vi "calculateSpectra.vi"(8 "ErrorIn":errorcluster, 10 "Tacho signal In":waveform(dbl), 11 "AccelerationDataIn":waveform(dbl)[](array[waveform])) -> (0 "ErrorOut":errorcluster, 1 "Rotational speed [RPM]":dbl format="%0.2f", 2 "AccelerationDataFrames":T8, 3 "AccelerationDataOut":waveform(dbl)[](array[waveform]), 4 "order power spectra":T7(array[cluster]) {"order 0" format="%.2p"; "delta order" format="%.2p"; "magnitude" format="%.2f"}, 5 "Tacho signal out":waveform(dbl), 6 "spectrum info":T1[](array[typedef]) {"x-axis units" items=["Time (s)"=0, "Frequency-CB (Hz)"=1, "Frequency-CPB (Hz)"=1248, "Frequency-Arbitrary (Hz)"=2357, "Quefrency (s)"=2, "Revolutions (rev)"=3, "Order"=4, "Speed (RPM)"=11, "Speed (rad/s)"=21, "Index"=65535]; "weighting filter" items=["Linear", "A-weighting", "B-weighting", "C-weighting", "ITU-R 468-4", "Dolby", "CCITT", "C-message", "Wb", "Wc", "Wd", "We", "Wf", "Wh", "Wj", "Wk", "Wm", "AES17 20 kHz lowpass", "AES17 40 kHz lowpass", "AES17 20 kHz highpass", "AES17 40 kHz highpass"]; "dB reference [EU]" format="%.2f"; "engineering units" items=["custom..."=0, "V"=1, "A"=21, "C"=30, "pC"=31, "s"=32, "-"=29, "Pa"=2, "N"=20, "g"=3, "m/s^2"=4, "m/s"=5, "m"=6, "mm/s"=12, "mm"=13, "micron/s"=14, "micron"=15, "in/s^2"=7, "in/s"=8, "in"=9, "mil/s"=10, "mil"=11, "rad/s^2"=16, "rad/s"=17, "rad"=18, "deg/s^2"=26, "deg/s"=27, "deg"=28, "RPM"=22, "cycle/s^2"=23, "Hz"=24, "cycle"=25, "strain"=19]; "spectral info"."window" items=["None "=0, "Hanning"=1, "Hamming"=2, "Blackman-Harris"=3, "Exact Blackman"=4, "Blackman"=5, "Flat Top"=6, "4 Term B-Harris "=7, "7 Term B-Harris"=8, "Low Sidelobe"=9, "Force - Exponential"=10, "Gaussian"=62]})   [LabVIEW 2019]
uses:
  AccelerationDataFrames.ctl
  <vilib>/addons/_NISVFA/_Shared subVIs/Controls/svc_Spectrum Info.ctl
  <vilib>/addons/_NISVFA/_Shared subVIs/Controls/svc_X-Axis Units.ctl
  <vilib>/addons/_NISVFA/_Shared subVIs/Controls/svc_Spectrum Type.ctl
  <vilib>/addons/_NISVFA/_Shared subVIs/Controls/svc_Engineering Units Text Ring.ctl
  <vilib>/addons/_NISVFA/_Shared subVIs/Controls/svc_Weighting Filter Text Ring.ctl
  <vilib>/addons/_NISVFA/_Shared subVIs/Controls/svc_Complimentary Spectrum Units.ctl
  <vilib>/addons/Sound and Vibration/svt_Calibration/SVL Scale Voltage to EU (1 Ch).vi
  <vilib>/Analysis/baseanly.llb/Mean (DBL).vi
  <vilib>/addons/Sound and Vibration/svt_Calibration/SVL Scale Voltage to EU (N Ch - 1 Info).vi
  <vilib>/addons/_NISVFA/_Shared subVIs/Common/svc_Set SV Channel Info.vi
  <vilib>/addons/_NISVFA/_Shared subVIs/Common/svc_Set SV Channel Info (variant).vi
  <vilib>/addons/_NISVFA/_Shared subVIs/Common/SVL Set dB Reference (variant).vi
  <vilib>/Waveform/WDTOps.llb/WDT Waveform Duration DBL.vi
  <vilib>/Waveform/WDTOps.llb/WDT Get Waveform Subset DBL.vi
  <vilib>/measure/madcrms.llb/Basic Averaged DC-RMS for 1 Chan.vi
  <vilib>/measure/maspectr.llb/FFT Spectrum (Real-Im) for 1 Chan.vi
  <vilib>/addons/_NISVFA/_Shared subVIs/Common/svc_Engineering Units to Unit Label.vi
  <vilib>/addons/_NISVFA/_Shared subVIs/Common/svc_Compute Scale Factor to Convert V to EU.vi
  <vilib>/addons/_NISVFA/_Shared subVIs/Common/svc_Compute Scale Factor to Convert C to EU.vi
  <vilib>/addons/_NISVFA/_Shared subVIs/Common/svc_Set dB ref if Pascal.vi
  <vilib>/addons/_NISVFA/_Shared subVIs/Common/svc_Caller VI Returned in Error Source.vi
  <vilib>/addons/Sound and Vibration/Order Analysis/Tach Process/OAT Analog Tacho Process (1 Tacho).vi
  <vilib>/addons/Sound and Vibration/Order Analysis/Resample Order Tracking/OAT Convert to Even Angle Signal (N Channels).vi
  <vilib>/addons/Sound and Vibration/Order Analysis/Resample Order Tracking/OAT Order Power Spectrum (N Channels).vi
  <vilib>/measure/NI_MAPro.lvlib
  <vilib>/addons/Sound and Vibration/Order Analysis/Tach Process/SoundVib_TachProcess.lvlib
  <vilib>/addons/Sound and Vibration/Order Analysis/Resample Order Tracking/SoundVib_OrderTracking.lvlib
  <vilib>/Analysis/NI_AALBase.lvlib
  <vilib>/addons/Sound and Vibration/svt_Calibration/SoundVib_Calibration.lvlib
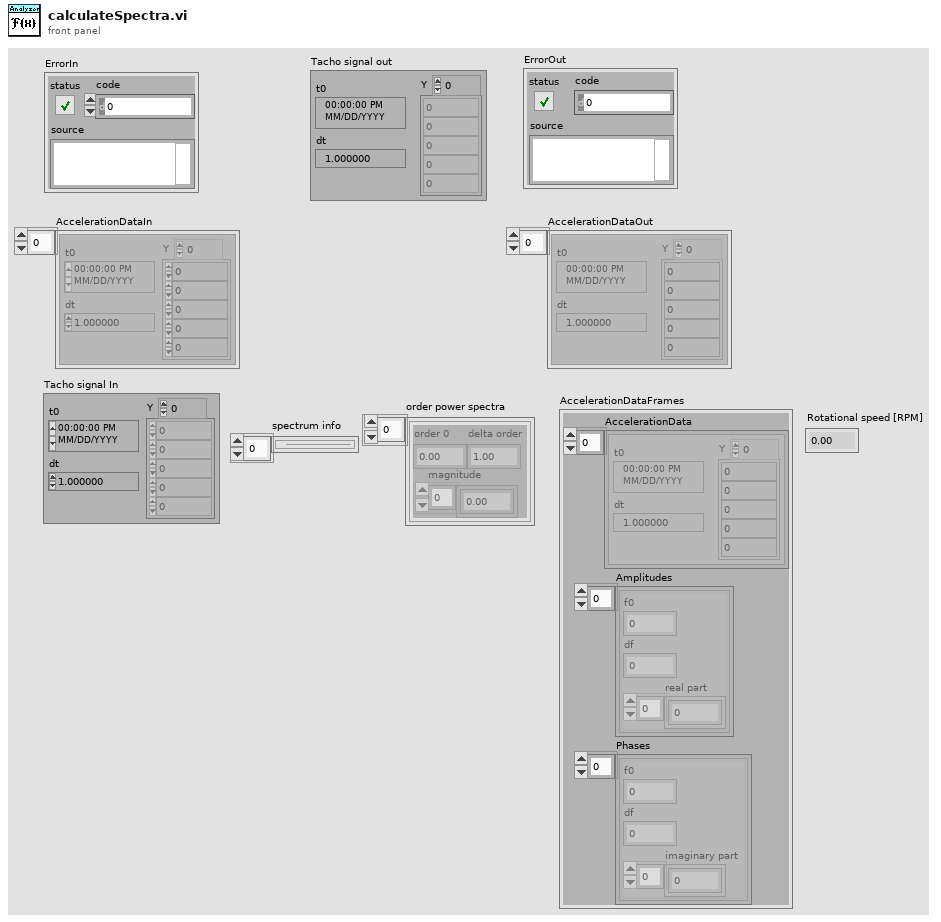
[diagram p1: front panel]
types:
  T1 = typedef "svc_Spectrum Info.ctl" = cluster{"channel name":string, "description":string, "x-axis units":T2, "spectral info":cluster{"spectrum type":T3, "linear/dB":enum16{"linear", "dB"}, "window":u16, "window size":i32, "FFT size":i32}, "engineering units":T4, "custom label":string, "dB reference [EU]":dbl, "peak units":enum16{"rms", "peak", "peak-peak"}, "weighting filter":T5, "spectral density?":bool, "unit label":string, "spectrum skewed?":bool, "complimentary spectrum units":T6}
  T2 = typedef "svc_X-Axis Units.ctl" = u16
  T3 = typedef "svc_Spectrum Type.ctl" = enum16{"FFT Spectrum [complex]", "Amplitude [Magnitude]", "Power [Magnitude^2]", "Cross Spectrum [complex]", "Frequency Response [Complex]"}
  T4 = typedef "svc_Engineering Units Text Ring.ctl" = u16
  T5 = typedef "svc_Weighting Filter Text Ring.ctl" = u16
  T6 = typedef "svc_Complimentary Spectrum Units.ctl" = enum16{"none", "radians", "degrees", "cycles", "imaginary"}
  T7 = cluster{"order 0":dbl, "delta order":dbl, "magnitude":dbl[]}[]
  T8 = typedef "AccelerationDataFrames.ctl" = cluster{"AccelerationData":waveform(dbl)[], "Amplitudes":cluster{"f0":dbl, "df":dbl, "real part":dbl[]}[], "Phases":cluster{"f0":dbl, "df":dbl, "imaginary part":dbl[]}[]}
  T9 = cluster{"averaging mode":enum16{"No averaging", "Vector averaging", "RMS averaging", "Peak hold"}, "weighting mode":enum16{"Linear", "Exponential"}, "number of averages":u32}
  T10 = enum16{"Rectangular (none)", "Hanning", "Low side lobe"}
  T11 = cluster{"f0":dbl, "df":dbl, "imaginary part":dbl[]}
  T12 = typedef "AnalyzerSettings.ctl" = cluster{"Create NS Timeout Code":i32, "Destroy NS Timeout Code":i32, "All threads":T13[], "Connected to app?":bool, "AnalysisSettings":T14}
  T13 = typedef "AThreads.ctl" = enum16{"UI", "analyzeAccelerationData", "aquireAccelerationData", "communicateWebServices", "TDMSmanager", "aquireTachoSignal"}
  T14 = typedef "AnalysisSettings.ctl" = cluster{"Fault Thresholds":T15, "Analysis series name":string, "Save data analysis?":bool, "Band size":i32, "OrderAnalysis?":bool, "Accelerometer":T17, "fs [Hz]":dbl, "Pulse per revolution":u16}
  T15 = typedef "Thresholds.ctl" = cluster{"Parameters labels":T16[], "Parameters thresholds":dbl[], "Freqs and thresholds":dbl[][], "Orders and thresholds":dbl[][]}
  T16 = typedef "FaultParameter.ctl" = enum16{"Kurtosis", "RMS", "Crest factor"}
  T17 = typedef "Accelerometer.ctl" = enum16{"None", "MPU6050", "MMA7351"}
  T18 = typedef "SoundVib_TachProcess.lvlib/speed profile.ctl" = cluster{"time [s]":dbl[], "speed [RPM]":dbl[]}
  T19 = typedef "svc_Resampled Channel Info.ctl" = cluster{"channel name":string, "description":string, " channel info":T20}
  T20 = typedef "svc_Channel Info.ctl" = cluster{"sensor sensitivity":dbl, "engineering units":T4, "dB reference":dbl, "custom label":string, "weighting filter":T5, "pregain":dbl}
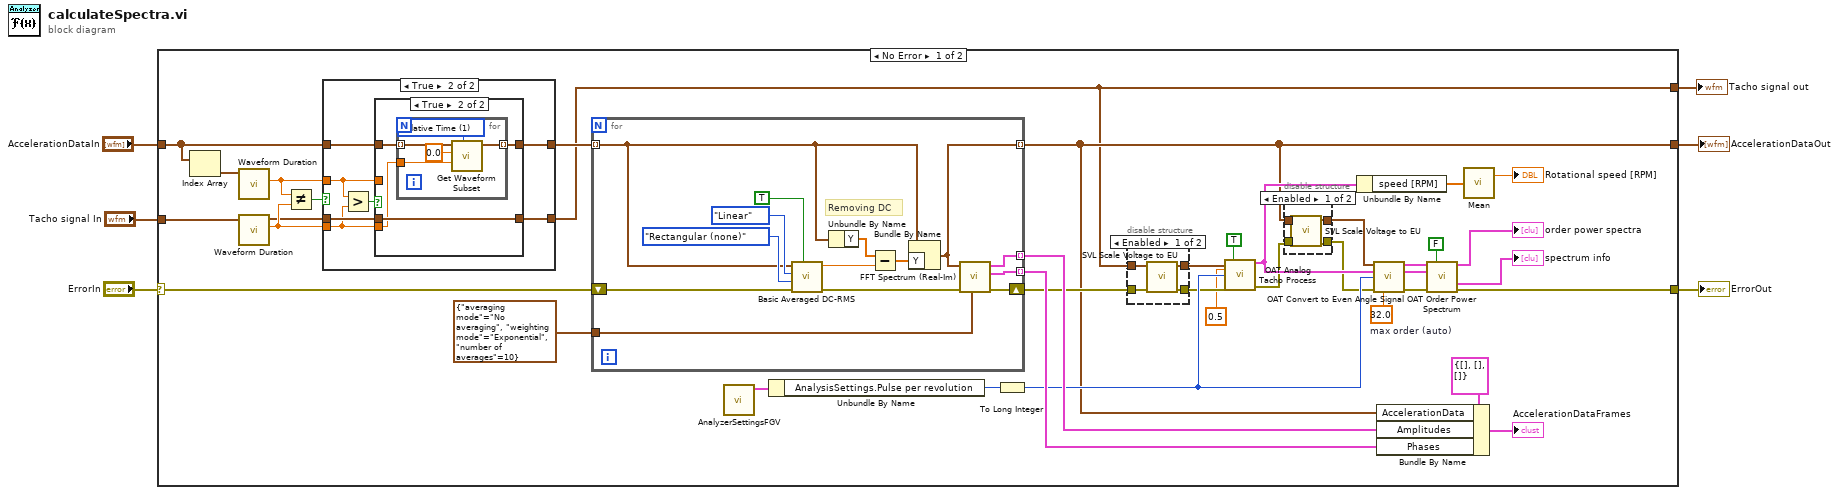
[diagram p0: block diagram]
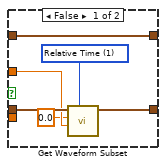
[diagram p5: hidden frame]
diagram:
  n1 = case shown="No Error" "ErrorIn" {
    selector: "ErrorIn" -> [w33 w97]
    tunnel: [w9 w97] -> w6
    tunnel: "AccelerationDataIn" -> [w34 w96]
    tunnel: [w10 w96] -> w3
    tunnel: "Tacho signal In" -> [w32 w95]
    tunnel: [w7 w95] -> w1
    frame No Error {
      w15 = 32.0  # max order (auto)
      n2 = Index Array(array=w34) -> (element=w35:waveform(dbl))  [unwired: 1 in]
      n3 = call-poly <vilib>:"Waveform Duration.vi"("waveform in"=w35) -> ("duration"=w38:dbl)  [unwired: 8 in, 2 out]
      n4 = call-poly <vilib>:"Waveform Duration.vi"("waveform in"=w32) -> ("duration"=w39:dbl, "waveform out"=w37:waveform(dbl))  [unwired: 8 in, 1 out]
      n5 = Not Equal?(x=w38, y=w39) -> (x != y?=w36:bool)
      n6 = case shown="True" w36 {
        tunnel: w34 -> [w58 w63]
        tunnel: w37 -> [w57 w64]
        tunnel: [w58 w59] -> w31
        tunnel: [w57 w60] -> w7
        tunnel: w38 -> [_ w62]
        tunnel: w39 -> [_ w61]
        frame False {
        }
        frame True {
          n7 = Greater?(x=w62, y=w61) -> (0:w65:bool)
          n8 = case shown="True" w65 {
            tunnel: w64 -> [w71 w75]
            tunnel: w63 -> [w68 w74]
            tunnel: w62 -> [w70 _]
            tunnel: w61 -> [_ w73]
            tunnel: [w69 w75] -> w60
            tunnel: [w68 w72] -> w59
            frame False {
              w66 = u16 1 items=["Samples", "Relative Time"] ("start/duration format")
              n9 = call-poly <vilib>:"Get Waveform Subset.vi"("start/duration format"=w66, "duration"=w70, "start samples/time"=0.0, "waveform in"=w71) -> ("waveform out"=w69:waveform(dbl))  [unwired: 2 in, 3 out]
            }
            frame True {
              n10 = for {
                tunnel: w74 -> [w80] mode=indexing
                tunnel: w73 -> [w79]
                tunnel: [w78] -> w72 mode=indexing
                w76 = u16 1 items=["Samples", "Relative Time"] ("start/duration format")
                n11 = call-poly <vilib>:"Get Waveform Subset.vi"("start/duration format"=w76, "duration"=w79, "start samples/time"=0.0, "waveform in"=w80) -> ("waveform out"=w78:waveform(dbl))  [unwired: 2 in, 3 out]
              }
            }
          }
        }
      }
      n12 = for {
        shift-right: [w94] -> w12
        shift-left: w33 -> [w90]
        tunnel: T9 {"averaging mode"=enum."No averaging", "weighting mode"=enum."Exponential", "number of averages"=10} ("averaging parameters") -> [w93]
        tunnel: [w92] -> w42 mode=indexing
        tunnel: [w91] -> w41 mode=indexing
        tunnel: w31 -> [w83] mode=indexing
        tunnel: [w81] -> w10 mode=indexing
        # "Removing DC"
        n13 = call-poly <vilib>:"Basic Averaged DC-RMS.vi"("reset"=TRUE, "error in (no error)"=w90, "window"=T10."Rectangular (none)", "averaging type"=enum16{"Linear", "Exponential"}."Linear", "signal in"=w83) -> ("error out"=w84:errorcluster, "DC value"=w86:dbl)  [unwired: 3 in, 2 out]
        n14 = Unbundle By Name(w83) -> ("Y"=w85:dbl[])
        n15 = Subtract(x=w85, y=w86) -> (x-y=w82:dbl[])
        n16 = Bundle By Name(cluster=w83, "Y"=w82) -> (w81:waveform(dbl))
        n17 = call-poly <vilib>:"FFT Spectrum (Real-Im).vi"("averaging parameters"=w93, "error in (no error)"=w84, "time signal"=w81) -> ("error out"=w94:errorcluster, "imaginary part"=w91:T11, "real part"=w92:cluster{"f0":dbl, "df":dbl, "real part":dbl[]})  [unwired: 4 in, 2 out]
      }
      n18 = call "AnalyzerSettingsFGV.vi"() -> ("AnalyzerSettingsOut"=w20:T12)  [unwired: 11 in]
      n19 = Unbundle By Name(w20) -> ("AnalysisSettings.Pulse per revolution"=w29:u16)
      n20 = To Long Integer(number=w29) -> (32bit integer=w30:i32)
      n21 = disable-structure shown="Enabled" {
        disable-tunnel: [w54 w56] -> w11
        disable-tunnel: [w53 w55] -> w19
        disable-tunnel: w7 -> [w52 w56]
        disable-tunnel: w12 -> [w51 w55]
        frame Enabled {
          n22 = call-poly <vilib>:"SVL Scale Voltage to EU.vi"("error in (no error)"=w51, "signal [V]"=w52) -> ("error out"=w53:errorcluster, "scaled signal [EU]"=w54:waveform(dbl))  [unwired: 7 in, 1 out]
        }
        frame Disabled {
        }
      }
      n23 = call-poly <vilib>:"OAT Analog Tacho Process.vi"("analog tacho signal"=w11, "missing pulses? (no:F)"=TRUE, "threshold (auto)"=0.5, "pulse/revolution (1)"=w30, "error in (no error)"=w19) -> ("speed profile"=w26:T18, "error out"=w24:errorcluster)  [unwired: 6 in, 3 out]
      n24 = disable-structure shown="Enabled" {
        disable-tunnel: [w48 w50] -> w23
        disable-tunnel: w10 -> [w47 w50]
        disable-tunnel: w24 -> [w46 w49]
        disable-tunnel: [w45 w49] -> w25
        frame Enabled {
          n25 = call-poly <vilib>:"SVL Scale Voltage to EU.vi"("error in (no error)"=w46, "signals [V]"=w47) -> ("error out"=w45:errorcluster, "scaled signals [EU]"=w48:waveform(dbl)[])  [unwired: 7 in, 1 out]
        }
        frame Disabled {
        }
      }
      n26 = Unbundle By Name(w26) -> ("speed [RPM]"=w27:dbl[])
      n27 = call-poly <vilib>:"OAT Convert to Even Angle Signal.vi"("scaled signals [EU]"=w23, "speed profile"=w26, "pulse/revolution (1)"=w30, "error in (no error)"=w25, "max order (auto)"=w15) -> ("even-angle signals"=w21:cluster{"r0":dbl, "dr":dbl, "Y":dbl[]}[], "even-angle channel info"=w18:T19[], "error out"=w17:errorcluster)  [unwired: 6 in, 2 out]
      n28 = Bundle By Name(cluster=T8 {"AccelerationData"=[], "Amplitudes"=[], "Phases"=[]} ("AccelerationDataFrames"), "AccelerationData"=w10, "Amplitudes"=w42, "Phases"=w41) -> (→"AccelerationDataFrames":T8)
      n29 = call-poly <vilib>:"OAT Order Power Spectrum.vi"("even-angle signals"=w21, "dB on? (T)"=FALSE, "even-angle channel info"=w18, "error in (no error)"=w17) -> ("order power spectra"=→"order power spectra":T7, "spectrum info"=→"spectrum info":T1[], "error out"=w9:errorcluster)  [unwired: 5 in, 4 out]
      n30 = call-poly <vilib>:"Mean.vi"("X"=w27) -> ("mean"=→"Rotational speed [RPM]":dbl)  [unwired: 1 out]
    }
    frame Error {
    }
  }
  "ErrorOut" <- w6
  "AccelerationDataOut" <- w3
  "Tacho signal out" <- w1
